vi "Actor Core.vi"(8 "error in":errorcluster, 11 "Synchronization Device in":refnum<class "NI DAQ.lvclass">) -> (0 "error out":errorcluster, 3 "Actor out":refnum<class "Actor.lvclass">)   [LabVIEW 2023, in "NI DAQ.lvlib" / "NI DAQ.lvclass"]
doc: "(<B>Filename</B>: Actor Framework.lvlib:Actor.lvclass:Actor Core.vi)\n\nReceives messages to the actor, reacts to them, and initiates any error handling that may shut the actor down.\n\nDescendant classes may override this VI to append parallel tasks for the actor to complete while it handles messages. Overrides use the Call Parent Method node."
uses:
  NI DAQ.lvclass
  C:/Program Files/National Instruments/LabVIEW 2023/vi.lib/ActorFramework/Actor/Actor.lvclass
  <vilib>/ActorFramework/Actor/Actor.lvclass
  <vilib>/ActorFramework/Actor/Actor.lvclass/Actor.ctl
  NI DAQ.lvclass/NI DAQ.ctl
  <vilib>/DAQmx/write.llb/DAQmx Write (Digital 1D Bool 1Chan 1Samp).vi
  <vilib>/DAQmx/miscellaneous.llb/DAQmx Fill In Error Info.vi
  Sync Device/Sync Device.lvclass
  NI DAQ.lvlib
panel:
  in  "Stop Button":bool
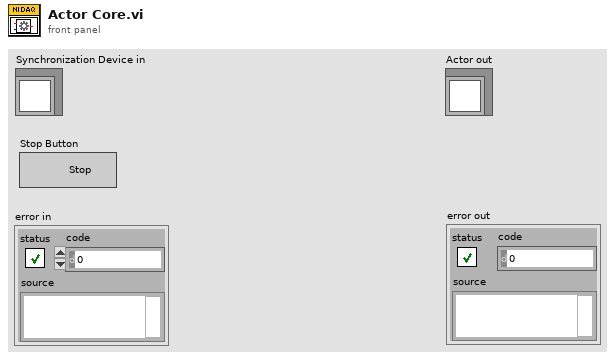
[diagram p1: front panel]
types:
  T1 = typedef "sync device settings.ctl" = cluster{"Interval (ms)":dbl, "ALEX":bool, "Shutter Enable":bool[], "Stream":bool, "Duty Cycle":dbl, "fluidics trigger frame":u16, "Frames to Skip":u32, "Frames to Acquire":i32}
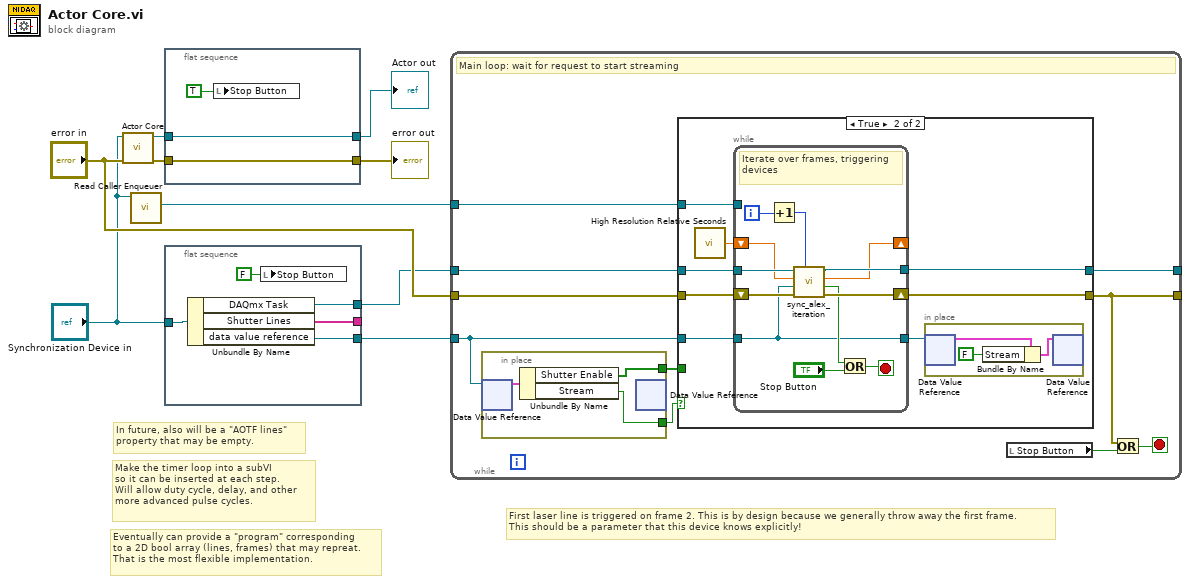
[diagram p0: block diagram]
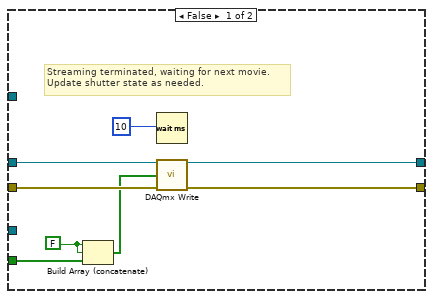
[diagram p2: hidden frame]
diagram:
  # "First laser line is triggered on frame 2. This is by design because we generally throw away the first frame.\nThis should be a parameter that this device knows explicitly!"
  # "Eventually can provide a \"program\" corresponding\nto a 2D bool array (lines, frames) that may repreat.\nThat is the most flexible implementation."
  # "Make the timer loop into a subVI\nso it can be inserted at each step.\nWill allow duty cycle, delay, and other\nmore advanced pulse cycles."
  # "In future, also will be a \"AOTF lines\"\nproperty that may be empty."
  n1 = call-parent "Actor Core.vi"("error in"="error in", "Device in"="Synchronization Device in") -> ("error out"=w6:errorcluster, "Actor out"=w9:refnum<class "Actor.lvclass">)  [unwired: 8 in]
  n2 = call <vilib>:"Read Caller Enqueuer.vi"("Actor"="Synchronization Device in") -> ("Caller Enqueuer"=w1:refnum<class "Message Enqueuer.lvclass">)  [unwired: 10 in]
  n3 = flat-sequence {
    tunnel: w9 -> [w12]
    tunnel: [w12] -> w8
    tunnel: [w11] -> w7
    tunnel: w6 -> [w11]
    frame #0 {
      n4 = local write "Stop Button"(TRUE) -> ()
    }
  }
  n5 = flat-sequence {
    tunnel: "Synchronization Device in" -> [w17]
    tunnel: [w16] -> _
    tunnel: [w15] -> w3
    tunnel: [w14] -> w4
    frame #0 {
      n6 = Unbundle By Name(w17) -> ("DAQmx Task"=w15:refnum<k21>, "Shutter Lines"=w16:string[], "data value reference"=w14:refnum<data-value>)
      n7 = local write "Stop Button"(FALSE ("Stop Button")) -> ()
    }
  }
  n8 = while {
    tunnel: w4 -> [w21]
    tunnel: w3 -> [w25]
    tunnel: [w26] -> _
    tunnel: "error in" -> [w27]
    tunnel: [w23] -> _
    tunnel: w1 -> [w18]
    stop <- w24 stop-if-true
    # "Main loop: wait for request to start streaming"
    n9 = in-place {
      in-place-border: [w29] -> w22
      in-place-border: [w28] -> w20
      n10 = in-place-dvr #1(w21) -> (w30:T1)  [unwired: 1 out]
      n11 = Unbundle By Name(w30) -> ("Shutter Enable"=w28:bool[], "Stream"=w29:bool)
      n12 = in-place-dvr #1() -> ()  [unwired: 1 in, 2 out]
    }
    n13 = case shown="True" w22 {
      tunnel: w27 -> [w36 w43]
      tunnel: [w38 w45] -> w26
      tunnel: w21 -> [_ w42]
      tunnel: w25 -> [w35 w44]
      tunnel: [w37 w39] -> w23
      tunnel: w20 -> [w33 _]
      tunnel: w18 -> [_ w41]
      frame False {
        w31 = FALSE
        # "Streaming terminated, waiting for next movie.\nUpdate shutter state as needed."
        n14 = Build Array (concatenate)(w31, w31, w33) -> (w34:bool[])
        n15 = Wait (ms)(milliseconds to wait=u32 10 ("millisecond multiple")) -> ()  [unwired: 1 out]
        n16 = call-poly <vilib>:"DAQmx Write.vi"("task/channels in"=w35, "data"=w34, "error in"=w36) -> ("task out"=w38:refnum<k21>, "error out"=w37:errorcluster)  [unwired: 10 in, 1 out]
      }
      frame True {
        n17 = call <vilib>:"High Resolution Relative Seconds.vi"() -> ("relative seconds"=w46:dbl)
        n18 = while {
          tunnel: w44 -> [w58]
          tunnel: [w60] -> w45
          shift-right: [w59] -> _
          shift-left: w46 -> [w53]
          tunnel: w42 -> [w50]
          tunnel: w41 -> [_]
          shift-right: [w61] -> w39
          shift-left: w43 -> [w57]
          tunnel: [w50] -> w40
          i -> [w52]
          stop <- w56 stop-if-true
          # "Iterate over frames, triggering devices"
          n19 = Increment(x=w52) -> (x+1=w51:i32)
          n20 = call "sync_alex_iteration.vi"("frame number\n(starts with 1)"=w51, "error in"=w57, "data value reference"=w50, "last frame (s)"=w53, "DAQmx Task"=w58) -> ("error out"=w61:errorcluster, "Stop?"=w54:bool, "relative seconds 2"=w59:dbl, "task out"=w60:refnum<k21>)  [unwired: 1 in]
          n21 = Or(x=w54, y="Stop Button") -> (x .or. y?=w56:bool)
        }
        n22 = in-place {
          n23 = in-place-dvr #2(w40) -> (w49:T1)  [unwired: 1 out]
          n24 = Bundle By Name(cluster=w49, "Stream"=FALSE) -> (w48:T1)
          n25 = in-place-dvr #2(w48) -> ()  [unwired: 2 out]
        }
      }
    }
    n26 = local read "Stop Button"() -> (w19:bool)
    n27 = Or(x=w23, y=w19) -> (x .or. y?=w24:bool)
  }
  "error out" <- w7
  "Actor out" <- w8
